vi "DB Fetch UI List.vi"(0 "Refnum in":T4, 1 "Identifier":string, 5 "UI List Type":T3, 7 "UI Device Type":T2, 9 "Measurement Role":T1, 11 "error in (no error)":errorcluster) -> (4 "Refnum out":T4, 6 "1D Results":string[](array[string]), 10 "2D Results":string[][](array[string]), 15 "error out":errorcluster)   [LabVIEW 2026, in "Database.lvlib"]
uses:
  Database.lvlib
  <vilib>/addons/database/Connection.llb/Conn ObjectReference.ctl
  controls/UI/UI List Type.ctl
  controls/UI/UI Device Type.ctl
  controls/UI/Measurement Role.ctl
  <vilib>/addons/database/Connection.llb/Conn Execute.vi
  <vilib>/addons/database/Recordset.llb/Rec Fetch Recordset Data (R).vi
  <vilib>/addons/database/Recordset.llb/Rec Destroy - Connection.vi
  <vilib>/addons/database/NI_Database_API.lvlib
  Settings/Settings.lvlib
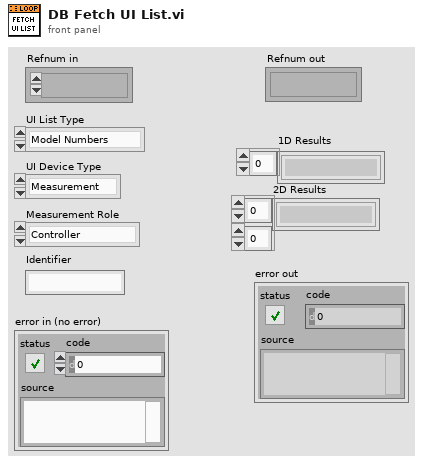
[diagram p1: front panel]
types:
  T1 = typedef "Settings.lvlib/Measurement Role.ctl" = enum16{"Controller", "Reference", "UUT", "Disable", "All"}
  T2 = typedef "Settings.lvlib/UI Device Type.ctl" = enum16{"Measurement", "Controller"}
  T3 = typedef "UI List Type.ctl" = enum16{"Model Numbers", "Serial Numbers", "Operators", "Calibration Points", "Start Run Times"}
  T4 = typedef "NI_Database_API.lvlib/Conn ObjectReference.ctl" = refnum<k1>
  T5 = typedef "NI_Database_API.lvlib/Rec ObjectReference.ctl" = refnum<k1>
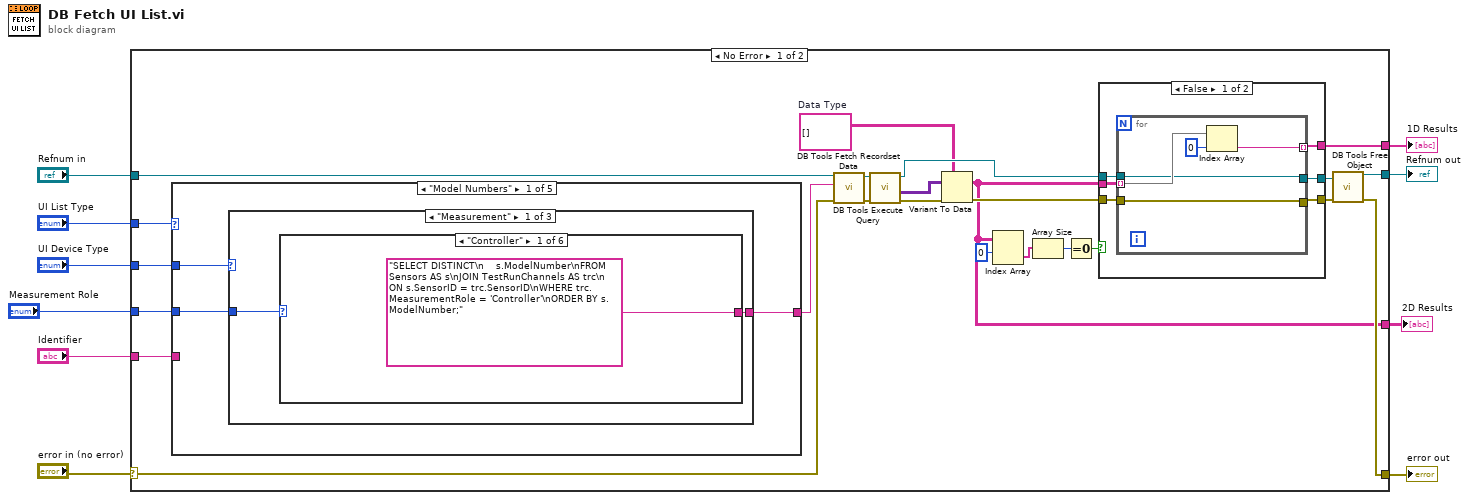
[diagram p0: block diagram]
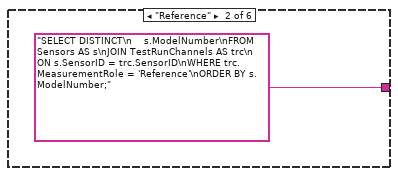
[diagram p2: hidden frame]
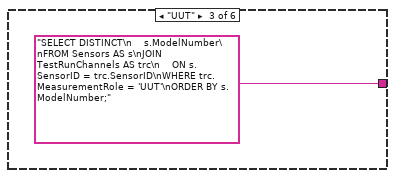
[diagram p3: hidden frame]
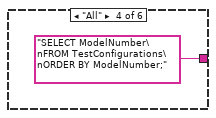
[diagram p4: hidden frame]
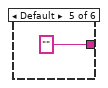
[diagram p5: hidden frame]
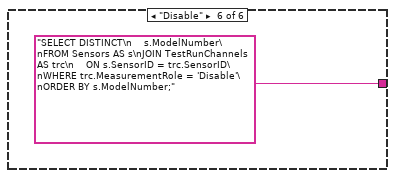
[diagram p6: hidden frame]
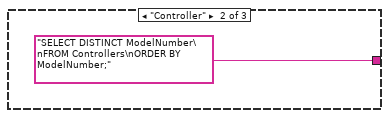
[diagram p7: hidden frame]
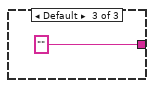
[diagram p8: hidden frame]
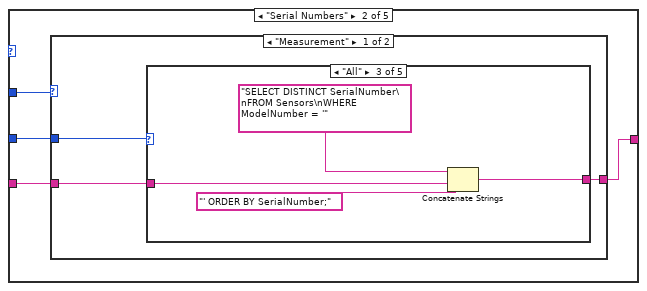
[diagram p9: hidden frame]
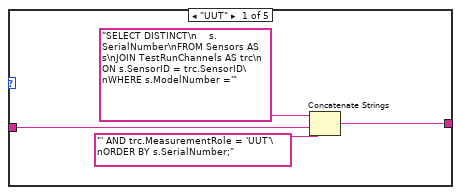
[diagram p10: hidden frame]
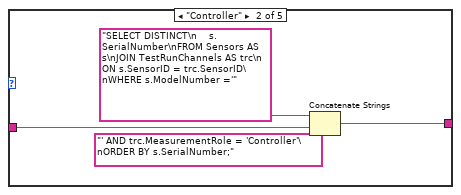
[diagram p11: hidden frame]
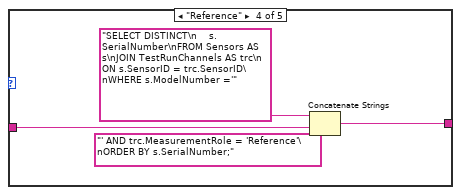
[diagram p12: hidden frame]
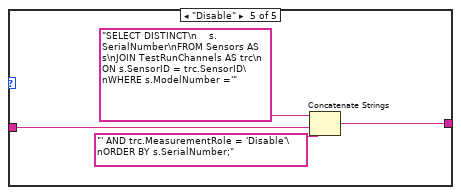
[diagram p13: hidden frame]
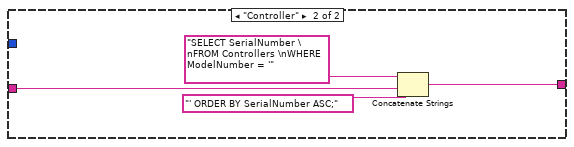
[diagram p14: hidden frame]
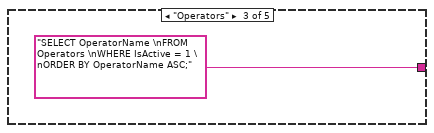
[diagram p15: hidden frame]
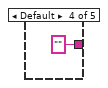
[diagram p16: hidden frame]
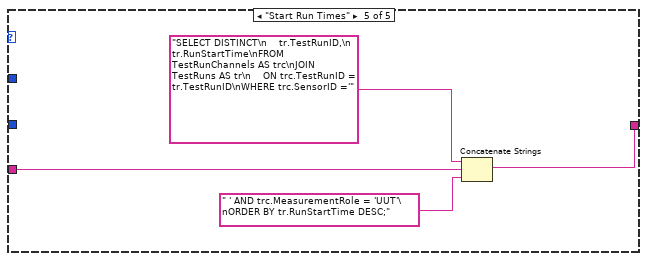
[diagram p17: hidden frame]
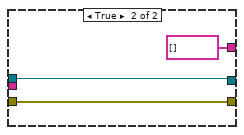
[diagram p18: hidden frame]
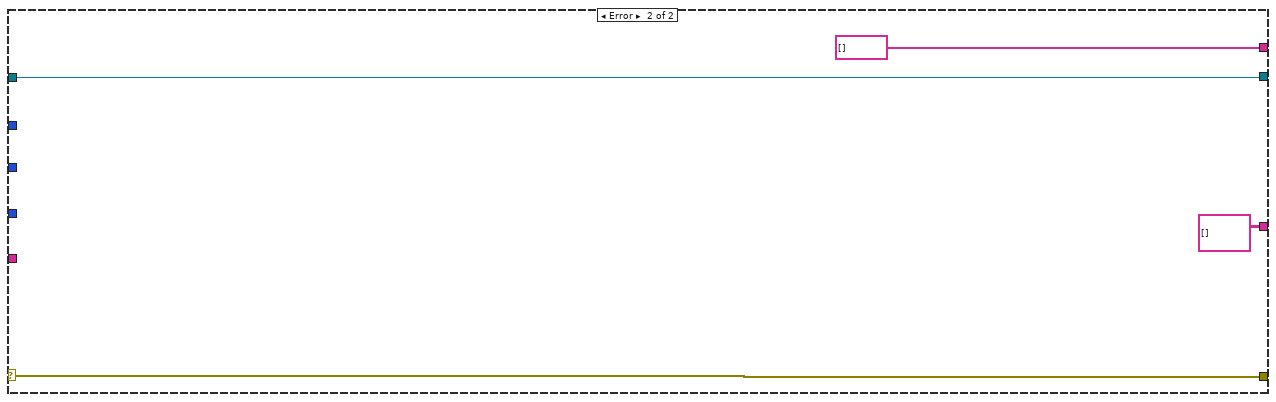
[diagram p19: hidden frame]
diagram:
  n1 = case shown="No Error" "error in (no error)" {
    selector: "error in (no error)" -> [w22 w102]
    tunnel: [w34 string[] []] -> w6
    tunnel: [w33 w101] -> w10
    tunnel: [w24 w102] -> w9
    tunnel: "Refnum in" -> [w23 w101]
    tunnel: "UI List Type" -> [w17 _]
    tunnel: "Identifier" -> [w14 _]
    tunnel: "UI Device Type" -> [w13 _]
    tunnel: [w12 string[][] [] ("Data Type")] -> w2
    tunnel: "Measurement Role" -> [w11 _]
    frame No Error {
      w15 = string[][] []  # Data Type
      n2 = case shown="\"Model Numbers\"" w17 {
        tunnel: [w37 w50 "SELECT OperatorName \nFROM Operators \nWHERE IsActive = 1 \nORDER BY OperatorName ASC;" "" w83] -> w16
        tunnel: w14 -> [_ w51 _ _ w84]
        tunnel: w13 -> [w36 w49 _ _ _]
        tunnel: w11 -> [w35 w48 _ _ _]
        frame "Model Numbers" {
          n3 = case shown="\"Measurement\"" w36 {
            tunnel: [w39 "SELECT DISTINCT ModelNumber\nFROM Controllers\nORDER BY ModelNumber;" ""] -> w37
            tunnel: w35 -> [w38 _ _]
            frame "Measurement" {
              n4 = case shown="\"Controller\"" w38 {
                tunnel: ["SELECT DISTINCT\n    s.ModelNumber\nFROM Sensors AS s\nJOIN TestRunChannels AS trc\n    ON s.SensorID = trc.SensorID\nWHERE trc.MeasurementRole = 'Controller'\nORDER BY s.ModelNumber;" "SELECT DISTINCT\n    s.ModelNumber\nFROM Sensors AS s\nJOIN TestRunChannels AS trc\n    ON s.SensorID = trc.SensorID\nWHERE trc.MeasurementRole = 'Reference'\nORDER BY s.ModelNumber;" "SELECT DISTINCT\n    s.ModelNumber\nFROM Sensors AS s\nJOIN TestRunChannels AS trc\n    ON s.SensorID = trc.SensorID\nWHERE trc.MeasurementRole = 'UUT'\nORDER BY s.ModelNumber;" "SELECT ModelNumber\nFROM TestConfigurations\nORDER BY ModelNumber;" "" "SELECT DISTINCT\n    s.ModelNumber\nFROM Sensors AS s\nJOIN TestRunChannels AS trc\n    ON s.SensorID = trc.SensorID\nWHERE trc.MeasurementRole = 'Disable'\nORDER BY s.ModelNumber;"] -> w39
                frame "Controller" {
                }
                frame "Reference" {
                }
                frame "UUT" {
                }
                frame "All" {
                }
                frame Default {
                }
                frame "Disable" {
                }
              }
            }
            frame "Controller" {
            }
            frame Default {
            }
          }
        }
        frame "Serial Numbers" {
          n5 = case shown="\"Measurement\"" w49 {
            tunnel: w51 -> [w54 w77]
            tunnel: [w53 w76] -> w50
            tunnel: w48 -> [w52 _]
            frame "Measurement" {
              n6 = case shown="\"All\"" w52 {
                tunnel: w54 -> [w57 w61 w65 w69 w73]
                tunnel: [w56 w60 w64 w68 w72] -> w53
                frame "UUT" {
                  n7 = Concatenate Strings("SELECT DISTINCT\n    s.SerialNumber\nFROM Sensors AS s\nJOIN TestRunChannels AS trc\n    ON s.SensorID = trc.SensorID\nWHERE s.ModelNumber ='", w57, "' AND trc.MeasurementRole = 'UUT'\nORDER BY s.SerialNumber;") -> (w56:string)
                }
                frame "Controller" {
                  n8 = Concatenate Strings("SELECT DISTINCT\n    s.SerialNumber\nFROM Sensors AS s\nJOIN TestRunChannels AS trc\n    ON s.SensorID = trc.SensorID\nWHERE s.ModelNumber ='", w61, "' AND trc.MeasurementRole = 'Controller'\nORDER BY s.SerialNumber;") -> (w60:string)
                }
                frame "All" {
                  n9 = Concatenate Strings("SELECT DISTINCT SerialNumber\nFROM Sensors\nWHERE ModelNumber = '", w65, "' ORDER BY SerialNumber;") -> (w64:string)
                }
                frame "Reference" {
                  n10 = Concatenate Strings("SELECT DISTINCT\n    s.SerialNumber\nFROM Sensors AS s\nJOIN TestRunChannels AS trc\n    ON s.SensorID = trc.SensorID\nWHERE s.ModelNumber ='", w69, "' AND trc.MeasurementRole = 'Reference'\nORDER BY s.SerialNumber;") -> (w68:string)
                }
                frame "Disable" {
                  n11 = Concatenate Strings("SELECT DISTINCT\n    s.SerialNumber\nFROM Sensors AS s\nJOIN TestRunChannels AS trc\n    ON s.SensorID = trc.SensorID\nWHERE s.ModelNumber ='", w73, "' AND trc.MeasurementRole = 'Disable'\nORDER BY s.SerialNumber;") -> (w72:string)
                }
              }
            }
            frame "Controller" {
              n12 = Concatenate Strings("SELECT SerialNumber \nFROM Controllers \nWHERE ModelNumber = '", w77, "' ORDER BY SerialNumber ASC;") -> (w76:string)
            }
          }
        }
        frame "Operators" {
        }
        frame Default {
        }
        frame "Start Run Times" {
          n13 = Concatenate Strings("SELECT DISTINCT\n    tr.TestRunID,\n    tr.RunStartTime\nFROM TestRunChannels AS trc\nJOIN TestRuns AS tr\n    ON trc.TestRunID = tr.TestRunID\nWHERE trc.SensorID ='", w84, " ' AND trc.MeasurementRole = 'UUT'\nORDER BY tr.RunStartTime DESC;") -> (w83:string)
        }
      }
      n14 = call-poly <vilib>:"DB Tools Execute Query.vi"("error in (no error)"=w22, "SQL query"=w16, "connection reference"=w23) -> ("error out"=w25:errorcluster, "recordset reference"=w26:T5)  [unwired: 5 in]
      n15 = call-poly <vilib>:"DB Tools Fetch Recordset Data.vi"("error in (no error)"=w25, "recordset reference"=w26) -> ("error out"=w27:errorcluster, "recordset data"=w28:variant[][], "recordset reference out"=w29:T5)  [unwired: 3 in]
      n16 = Variant To Data(error in=w27, type=w15, Variant=w28) -> (data=w12:string[][], error out=w30:errorcluster)
      n17 = Index Array(array=w12, index (row)=0) -> (element=w20:string[])  [unwired: 1 in]
      n18 = Array Size(array=w20) -> (size(s)=w19:i32)
      n19 = Equal To 0?(x=w19) -> (x = 0?=w18:bool)
      n20 = case shown="False" w18 {
        tunnel: [w90 string[] []] -> w34
        tunnel: w12 -> [w89 _]
        tunnel: [w88 w97] -> w32
        tunnel: [w87 w98] -> w31
        tunnel: w30 -> [w86 w97]
        tunnel: w29 -> [w85 w98]
        frame False {
          n21 = for {
            tunnel: w86 -> [w92]
            tunnel: w85 -> [w91]
            tunnel: w89 -> [w94] mode=indexing
            tunnel: [w93] -> w90 mode=indexing
            tunnel: [w91] -> w87
            tunnel: [w92] -> w88
            n22 = Index Array(array=w94, index=0) -> (element=w93:string)
          }
        }
        frame True {
        }
      }
      n23 = call-poly <vilib>:"DB Tools Free Object.vi"("error in (no error)"=w32, "recordset reference"=w31) -> ("error out"=w24:errorcluster, "connection reference"=w33:T4)  [unwired: 8 in]
    }
    frame Error {
    }
  }
  "Refnum out" <- w10
  "error out" <- w9
  "1D Results" <- w6
  "2D Results" <- w2
